vi "Init.vi"(8 "Queue Mailbox":refnum<data-value>, 9 "Queue Self":refnum<data-value>, 10 "Queue Self Alias":string) -> (3 "Base Queue jettl out":refnum<class "Base Queue jettl.lvclass">)   [LabVIEW 2021, in "jettl.lvlib" / "Base Queue jettl.lvlib" / "Base Queue jettl.lvclass"]
uses:
  Base Queue jettl.lvclass
  Queue Mailbox/Queue Mailbox/Queue Mailbox.lvclass
  Msg Strategy/Msg Strategy.lvclass
  State/Nominal State/Nominal State.lvclass
  C:/git/jettl/src/jettl/Base Queue jettl/State/State/State.lvclass
  Base Queue jettl.lvclass/Base Queue jettl.ctl
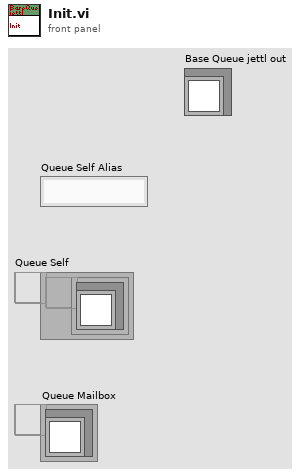
[diagram p1: front panel]
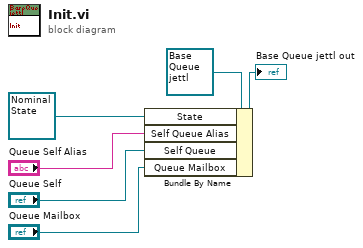
[diagram p0: block diagram]
diagram:
  n1 = Bundle By Name(cluster=refnum<class "Base Queue jettl.lvclass"> refnum ("Self Actor in"), "State"=refnum<class "Nominal State.lvclass"> refnum ("jettl.lvlib:Nominal Queue State.lvclass"), "Self Queue Alias"="Queue Self Alias", "Self Queue"="Queue Self", "Queue Mailbox"="Queue Mailbox") -> (→"Base Queue jettl out":refnum<class "Base Queue jettl.lvclass">)
